vi "Get Package Attributes (All Versions).vi"(8 "error in":errorcluster, 11 "package name":string) -> (0 "error out":errorcluster, 2 "package attributes (all versions)":T1[](array[typedef]), 3 "package name out":string)   [LabVIEW 2014, in "NIPM_API.lvlib"]
doc: "Returns the attributes for all versions of the specified package\n\nINPUT(s)\n<B>Package name</B>: Specifies the package\n\nOUTPUT(s)\n<B>Package name out</B>: Outputs the package name\n\n<B>Package attributes (all versions)</B>: Outputs a 1D array containing the package attributes for all versions of the specified package"
uses:
  NIPM_API.lvlib
  _support/package attributes.ctl
panel:
  out "cmd standard output":string
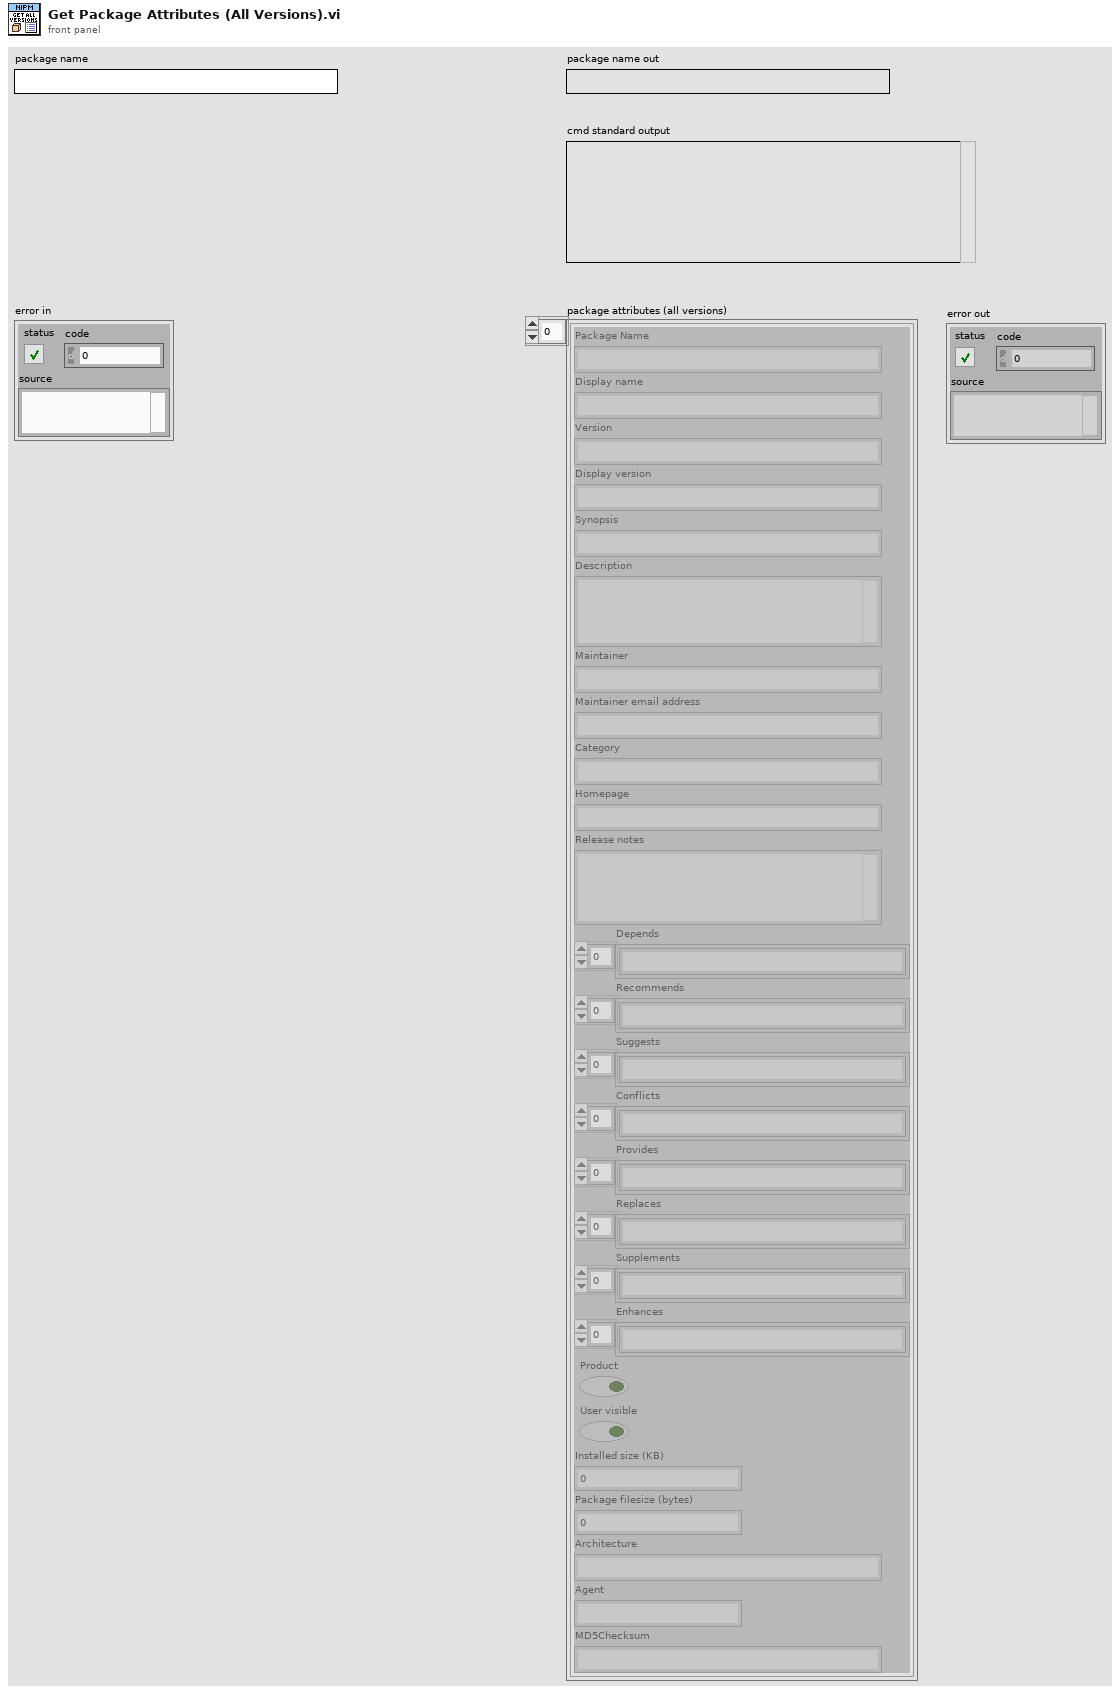
[diagram p1: front panel]
types:
  T1 = typedef "NIPM_API.lvlib/package attributes.ctl" = cluster{"Package Name":string, "Display name":string, "Version":string, "Display version":string, "Synopsis":string, "Description":string, "Maintainer":string, "Maintainer email address":string, "Category":string, "Homepage":string, "Release notes":string, "Depends":string[], "Recommends":string[], "Suggests":string[], "Conflicts":string[], "Provides":string[], "Replaces":string[], "Supplements":string[], "Enhances":string[], "Product":bool, "User visible":bool, "Installed size (KB)":u64, "Package filesize (bytes)":u64, "Architecture":string, "Agent":string, "MD5Checksum":string}
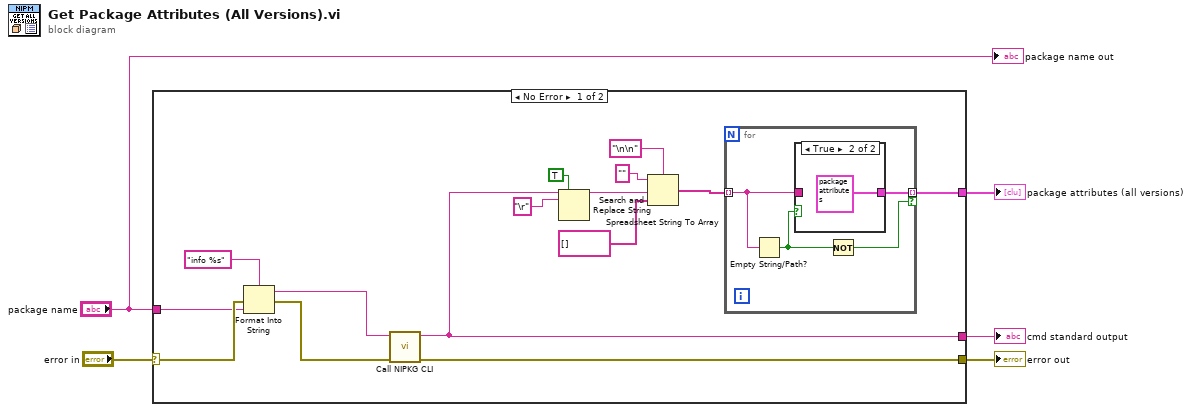
[diagram p0: block diagram]
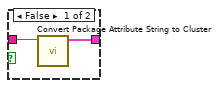
[diagram p2: hidden frame]
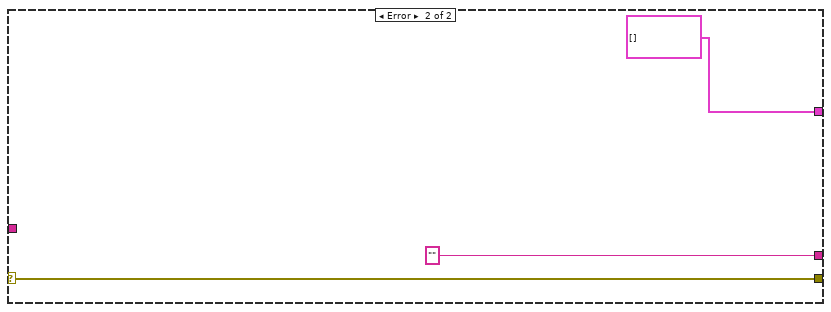
[diagram p3: hidden frame]
diagram:
  n1 = case shown="No Error" "error in" {
    selector: "error in" -> [w19 w30]
    tunnel: [w17 w30] -> w4
    tunnel: [w15 "" ("standard output")] -> w3
    tunnel: "package name" -> [w8 _]
    tunnel: [w6 T1[] []] -> w1
    frame No Error {
      n2 = Format Into String(format string="info %s", error in=w19, w8) -> (resulting string=w16:string, error out=w18:errorcluster)  [unwired: 1 in]
      n3 = call "Call NIPKG CLI.vi"("error in (no error)"=w18, "command"=w16) -> ("error out"=w17:errorcluster, "command line standard output"=w15:string)  [unwired: 8 in]
      n4 = Search and Replace String(replace all?=TRUE ("replace all? (F)"), input string=w15, search string="\r") -> (result string=w12:string)  [unwired: 5 in, 3 out]
      n5 = Spreadsheet String To Array(delimiter (Tab)="\n\n", format string="", spreadsheet string=w12, array type (2D Dbl)=string[] []) -> (array=w7:string[])
      n6 = for {
        tunnel: w7 -> [w23] mode=indexing
        tunnel: [w24] -> w6 mode=indexing if=w21
        n7 = Empty String/Path?(string/path=w23) -> (empty?=w22:bool)
        n8 = case shown="True" w22 {
          tunnel: [w26 T1 {"Package Name"="", "Display name"="", "Version"="", "Display version"="", "Synopsis"="", "Description"="", "Maintainer"="", "Maintainer email address"="", "Category"="", "Homepage"="", "Release notes"="", "Depends"=[], "Recommends"=[], "Suggests"=[], "Conflicts"=[], "Provides"=[], "Replaces"=[], "Supplements"=[], "Enhances"=[], "Product"=FALSE, "User visible"=FALSE, "Installed size (KB)"=0, "Package filesize (bytes)"=0, "Architecture"="", "Agent"="", "MD5Checksum"=""} ("package attributes")] -> w24
          tunnel: w23 -> [w25 _]
          frame False {
            n9 = call "Convert Package Attribute String to Cluster.vi"("package attributes string"=w25) -> ("package attributes"=w26:T1)  [unwired: 9 in, 1 out]
          }
          frame True {
          }
        }
        n10 = Not(x=w22) -> (.not. x?=w21:bool)
      }
    }
    frame Error {
    }
  }
  "error out" <- w4
  "cmd standard output" <- w3
  "package attributes (all versions)" <- w1
  "package name out" <- "package name"
